vi "Read IP.vi"(8 "error in (no error)":errorcluster, 11 "Ini File in":refnum<class "Ini File.lvclass">) -> (0 "error out":errorcluster, 2 "Read IP":string, 3 "Ini File out":refnum<class "Ini File.lvclass">)   [LabVIEW 2021, in "File Library.lvlib" / "Ini File.lvclass"]
uses:
  Ini File.lvclass
  Ini File.lvclass/Ini File.ctl
  <vilib>/Utility/config.llb/Read Key (String).vi
  <vilib>/Utility/config.llb/NI_LVConfig.lvlib
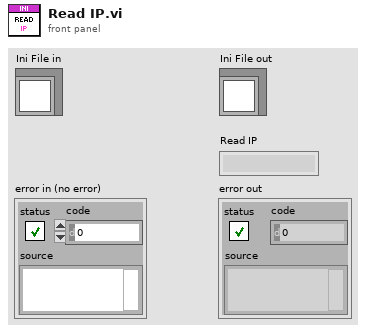
[diagram p1: front panel]
types:
  T1 = typedef "NI_LVConfig.lvlib/Config Data RefNum.ctl" = refnum<k1>
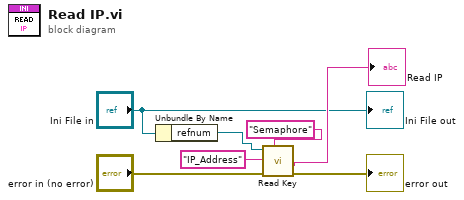
[diagram p0: block diagram]
diagram:
  n1 = Unbundle By Name("Ini File in") -> ("refnum"=w1:T1)
  n2 = call-poly <vilib>:"Read Key.vi"("section"="Semaphore", "error in (no error)"="error in (no error)", "key"="IP_Address" ("section"), "refnum"=w1) -> ("value"=→"Read IP":string)  [unwired: 4 in, 3 out]
  "error out" <- "error in (no error)"
  "Ini File out" <- "Ini File in"
